vi "Set Enable State on Multiple Controls.vi"(10 "Enable?":bool, 11 "Controls":refnum<vi>[](array[refnum])) -> (3 "Controls dup":refnum<vi>[](array[refnum]))   [LabVIEW 2021]
doc: "Enable or disable the 'Controls' based on 'Enable?'"
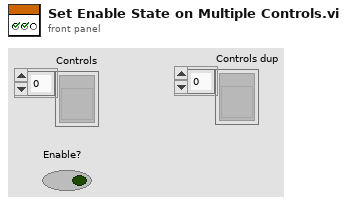
[diagram p1: front panel]
types:
  T1 = enum8{"Enabled", "Disabled", "Disabled and Grayed Out"}
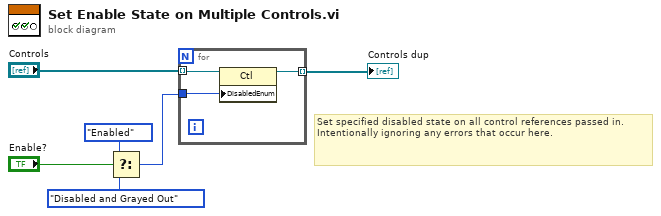
[diagram p0: block diagram]
diagram:
  # "Set specified disabled state on all control references passed in. Intentionally ignoring any errors that occur here."
  n1 = Select(t=T1."Enabled" ("Disabled"), s="Enable?", f=T1."Disabled and Grayed Out" ("Disabled")) -> (s? t:f=w4:T1)
  n2 = for {
    tunnel: "Controls" -> [w9] mode=indexing
    tunnel: w4 -> [w8]
    tunnel: [w7] -> w1 mode=indexing
    n3 = property class="Ctl"(reference=w9, "DisabledEnum"=w8) -> (reference out=w7:refnum<vi>)  [unwired: 1 in, 1 out]
  }
  "Controls dup" <- w1
